vi "CalcSystemState.vi"(1 "Motor States":T1[](array[typedef])) -> (0 "system state":T1)   [LabVIEW 2015]
uses:
  MotorStates.ctl
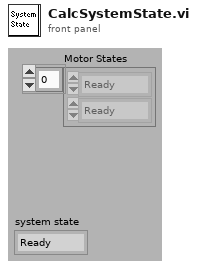
[diagram p1: front panel]
types:
  T1 = typedef "MotorStates.ctl" = enum16{"Ready", "Moving", "Uninitialized", "Error"}
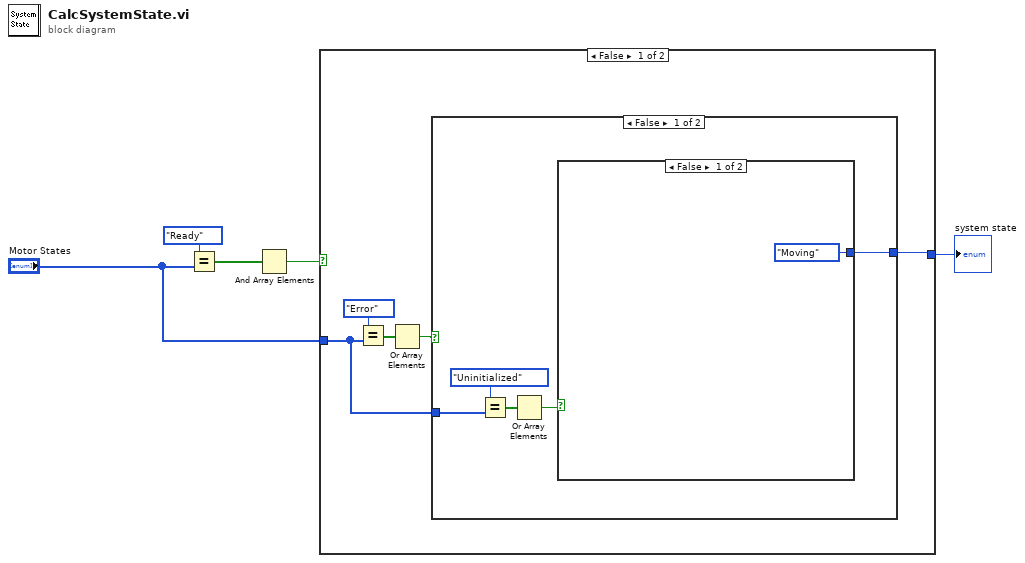
[diagram p0: block diagram]
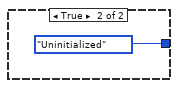
[diagram p2: hidden frame]
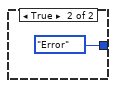
[diagram p3: hidden frame]
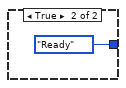
[diagram p4: hidden frame]
diagram:
  n1 = Equal?(x=MotorStates."Ready" ("GS State"), y="Motor States") -> (x = y?=w4:bool[])
  n2 = And Array Elements(Boolean array=w4) -> (logical AND=w3:bool)
  n3 = case shown="False" w3 {
    tunnel: [w9 MotorStates."Ready" ("GS State")] -> w2
    tunnel: "Motor States" -> [w8 _]
    frame False {
      n4 = Equal?(x=MotorStates."Error" ("GS State"), y=w8) -> (x = y?=w7:bool[])
      n5 = Or Array Elements(Boolean array=w7) -> (logical OR=w6:bool)
      n6 = case shown="False" w6 {
        tunnel: [w11 MotorStates."Error" ("GS State")] -> w9
        tunnel: w8 -> [w14 _]
        frame False {
          n7 = Equal?(x=MotorStates."Uninitialized" ("GS State"), y=w14) -> (x = y?=w13:bool[])
          n8 = Or Array Elements(Boolean array=w13) -> (logical OR=w12:bool)
          n9 = case shown="False" w12 {
            tunnel: [MotorStates."Moving" ("GS State") MotorStates."Uninitialized" ("GS State")] -> w11
            frame False {
            }
            frame True {
            }
          }
        }
        frame True {
        }
      }
    }
    frame True {
    }
  }
  "system state" <- w2
